vi "Validate Reference by Name.vi"(8 "error in":errorcluster, 10 "name":string, 11 "item in":T1 format="%.0x") -> (0 "error out":errorcluster, 3 "item out":T1 format="%.0x")   [LabVIEW 2020, in "Scan Engine Scripting.lvlib"]
uses:
  Scan Engine Scripting.lvlib
  <vilib>/NI VeriStand/Custom Device API/Custom Device Item Ref.ctl
  NationalInstruments.VeriStand.SystemDefinitionAPI
  Scan Engine Dependencies.llb/Error Strings.vi
  Scan Engine Dependencies.llb/Scan Engine Custom Device.lvlib
  <vilib>/NI VeriStand/Custom Device API/Custom Device API.lvlib
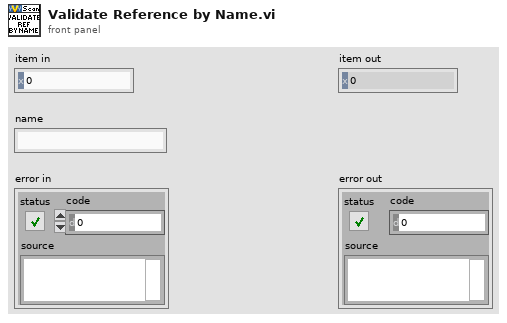
[diagram p1: front panel]
types:
  T1 = typedef "Custom Device API.lvlib/Custom Device Item Ref.ctl" = u64
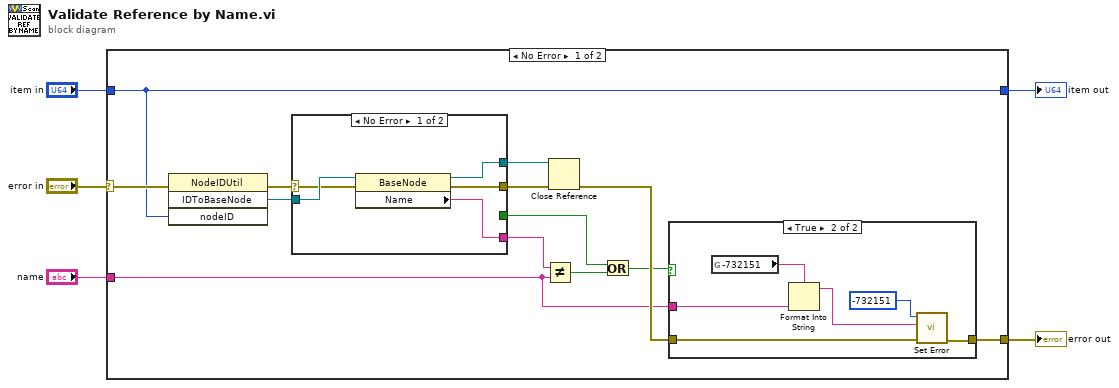
[diagram p0: block diagram]
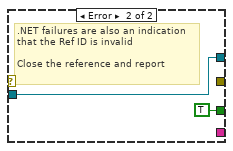
[diagram p2: hidden frame]
diagram:
  n1 = case shown="No Error" "error in" {
    selector: "error in" -> [w7 w33]
    tunnel: [w13 w33] -> w5
    tunnel: "name" -> [w12 _]
    tunnel: "item in" -> [w6 w34]
    tunnel: [w6 w34] -> w1
    frame No Error {
      n2 = invoke class="NodeIDUtil" method="IDToBaseNode"(error in=w7, "nodeID"=w6) -> (error out=w11:errorcluster, "IDToBaseNode"=w15:refnum<k24>)  [unwired: 2 in, 2 out]
      n3 = case shown="No Error" w11 {
        selector: w11 -> [w19 _]
        tunnel: [w23 _] -> w18
        tunnel: [w22 _] -> w17
        tunnel: [w21 w25] -> w16
        tunnel: w15 -> [w20 w25]
        tunnel: [_ TRUE] -> w9
        frame No Error {
          n4 = property class="BaseNode"(reference=w20, error in=w19) -> (reference out=w21:refnum<k24>, error out=w22:errorcluster, "Name"=w23:string)
        }
        frame Error {
          # ".NET failures are also an indication\nthat the Ref ID is invalid\n\nClose the reference and report"
        }
      }
      n5 = Not Equal?(x=w18, y=w12) -> (x != y?=w8:bool)
      n6 = Close Reference(reference=w16, error in (no error)=w17) -> (error out=w14:errorcluster)
      n7 = Or(x=w9, y=w8) -> (x .or. y?=w10:bool)
      n8 = case shown="True" w10 {
        tunnel: w14 -> [w26 w29]
        tunnel: [w26 w28] -> w13
        tunnel: w12 -> [_ w32]
        frame False {
        }
        frame True {
          n9 = global read "Error Strings.vi" "-732151"() -> (w27:string)
          n10 = Format Into String(format string=w27, w32) -> (resulting string=w31:string)  [unwired: 2 in, 1 out]
          n11 = call "Set Error.vi"("error in (no error)"=w29, "Message"=w31, "Code"=-732151 ("error code (0)")) -> ("error out"=w28:errorcluster)  [unwired: 8 in]
        }
      }
    }
    frame Error {
    }
  }
  "error out" <- w5
  "item out" <- w1
